vi "AlignFormOrigin.vi"(0 "This VI":refnum<vi>) -> ()   [LabVIEW 2024]
uses:
  <vilib>/Utility/miscctls.llb/LVPointTypeDef.ctl
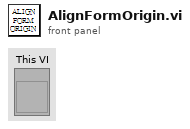
[diagram p1: front panel]
types:
  T1 = typedef "LVPointTypeDef.ctl" = cluster{"Horizontal":i16, "Vertical":i16}
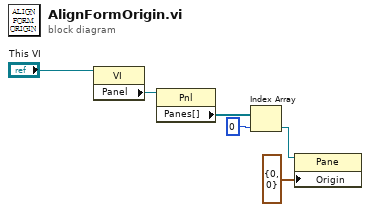
[diagram p0: block diagram]
diagram:
  n1 = property class="VI"(reference="This VI") -> ("Panel"=w6:refnum<vi>)  [unwired: 1 in, 2 out]
  n2 = property class="Pnl"(reference=w6) -> ("Panes[]"=w5:refnum<vi>[])  [unwired: 1 in, 2 out]
  n3 = Index Array(array=w5, index=0) -> (element=w3:refnum<vi>)
  n4 = property class="Pane"(reference=w3, "Origin"=T1 {"Horizontal"=0, "Vertical"=0}) -> ()  [unwired: 1 in, 2 out]
